vi "Enable Joystick Impl.vi"(8 "error in (no error)":errorcluster, 10 "Enable":bool, 11 "Nikon Ti2 Stage in":refnum<class "Nikon Ti2 Stage.lvclass">) -> (0 "error out":errorcluster, 3 "Nikon Ti2 Stage out":refnum<class "Nikon Ti2 Stage.lvclass">)   [LabVIEW 2023, in "Nikon Ti2 Stage.lvlib" / "Nikon Ti2 Stage.lvclass"]
uses:
  Nikon Ti2 Stage.lvclass
  Nikon Ti2 Stage.lvclass/Nikon Ti2 Stage.ctl
  Microscope/ti2lv/ti2lv.lvlib
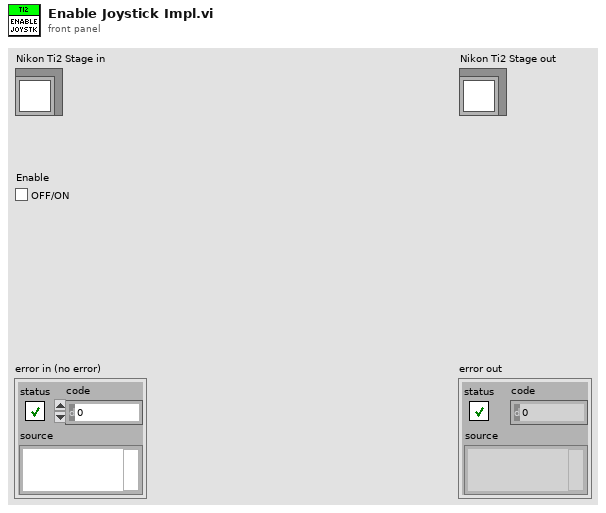
[diagram p1: front panel]
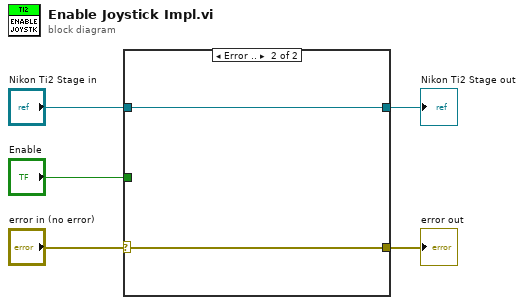
[diagram p0: block diagram]
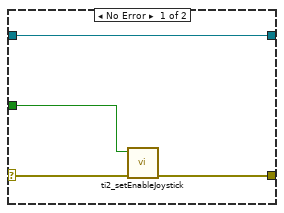
[diagram p2: hidden frame]
diagram:
  n1 = case shown="Error .." "error in (no error)" {
    selector: "error in (no error)" -> [w8 w10]
    tunnel: [w7 w10] -> w4
    tunnel: "Nikon Ti2 Stage in" -> [w9 w11]
    tunnel: [w9 w11] -> w2
    tunnel: "Enable" -> [w6 _]
    frame No Error {
      n2 = call "ti2_setEnableJoystick.vi"("error in (no error)"=w8, "value"=w6) -> ("error out"=w7:errorcluster)  [unwired: 9 in]
    }
    frame Error {
    }
  }
  "error out" <- w4
  "Nikon Ti2 Stage out" <- w2
